vi "ntitled 1.vi"() -> ()   [LabVIEW 2020]
panel:
  out "GRÁFICO DE LA SEÑAL":dynamicdata(graph)
  out "Alarma":bool
  in  "Lim":dbl
  in  "?":bool
  in  "Temp":dbl(slide) scale=0.0..100.0
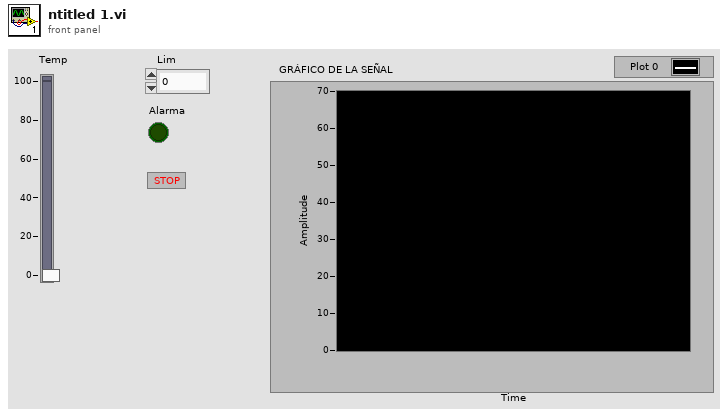
[diagram p1: front panel]
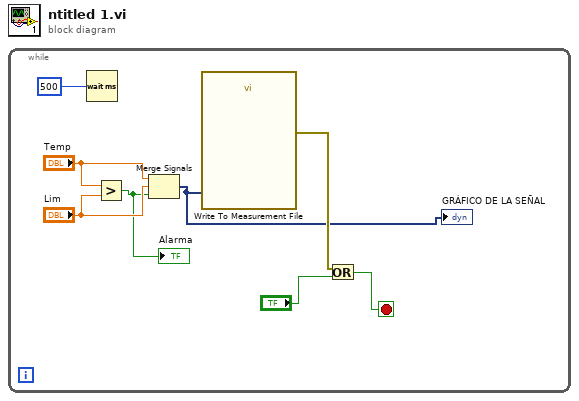
[diagram p0: block diagram]
diagram:
  n1 = while {
    stop <- w7 stop-if-true
    n2 = Wait (ms)(milliseconds to wait=500) -> ()  [unwired: 1 out]
    n3 = Greater?(x="Temp", y="Lim") -> (0:w2:bool)
    "Alarma" <- w2
    n4 = Merge Signals("Temp", "Lim", w2) -> (w1:dynamicdata)
    "GRÁFICO DE LA SEÑAL" <- w1
    n5 = call "Write To Measurement File"("Signals"=w1) -> ("error out"=w6:errorcluster)  [unwired: 16 in, 2 out]
    n6 = Or(x=w6, y="?") -> (x .or. y?=w7:bool)
  }
